vi "Write Response to Value Outside Limits.vi"(5 "Out of Range Action":T1, 9 "Numeric in":refnum<class "Numeric.lvclass">) -> (3 "Numeric out":refnum<class "Numeric.lvclass">)   [LabVIEW 2014, in "Raspberry Pi Compatible Compiler for LabVIEW.lvlib" / "Numeric.lvclass"]
uses:
  Numeric.lvclass
  <vilib>/Utility/miscctls.llb/LVOutOfRangeActionTypeDef.ctl
  Numeric.lvclass/Numeric.ctl
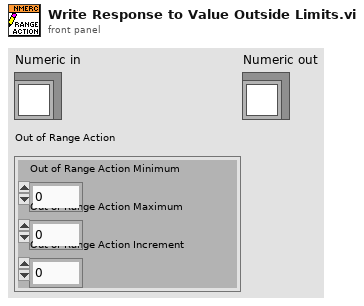
[diagram p1: front panel]
types:
  T1 = typedef "LVOutOfRangeActionTypeDef.ctl" = cluster{"Out of Range Action Minimum":u8, "Out of Range Action Maximum":u8, "Out of Range Action Increment":u8}
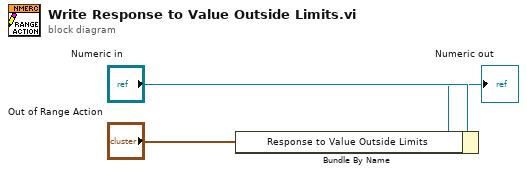
[diagram p0: block diagram]
diagram:
  n1 = Bundle By Name(cluster="Numeric in", "Response to Value Outside Limits"="Out of Range Action") -> (→"Numeric out":refnum<class "Numeric.lvclass">)
